vi "signal-NetVar-publisher.vi"() -> ()   [LabVIEW 2020]
uses:
  <vilib>/measure/NI_MABase.lvlib
panel:
  in  "Cluster":cluster{"Sampling Freq":dbl, "Samples":dbl}
  in  "Signal type":u16(ring) items=["Sine Wave", "Triangle Wave", "Square Wave", "Sawtooth Wave"]
  in  "Czestotliwosc":dbl(knob) scale=0.01..500.0
  in  "Amplituda":dbl(knob) scale=0.01..10.0
  in  "stop":bool
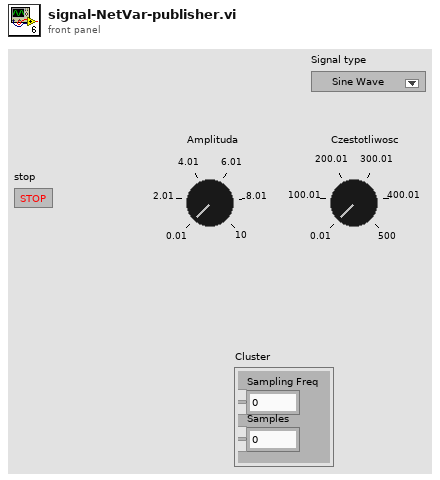
[diagram p1: front panel]
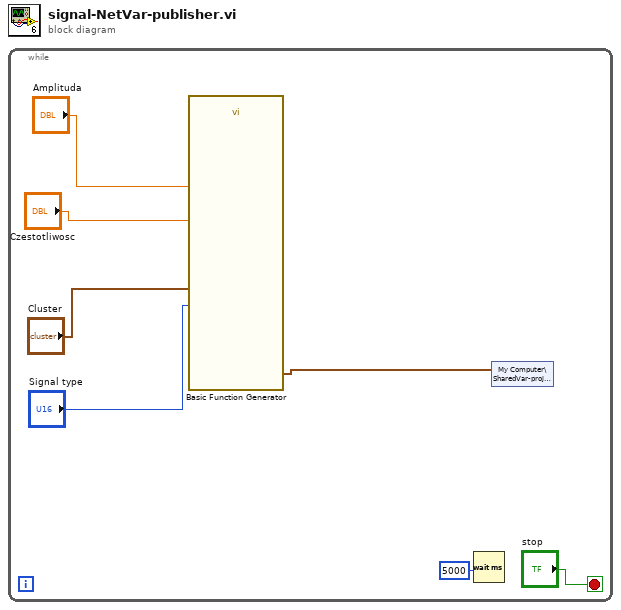
[diagram p0: block diagram]
diagram:
  n1 = while {
    stop <- "stop" stop-if-true
    n2 = call <vilib>:"Basic Function Generator.vi"("sampling info"="Cluster", "signal type"="Signal type", "amplitude"="Amplituda", "frequency"="Czestotliwosc") -> ("signal out"=w1:waveform(dbl))  [unwired: 5 in, 2 out]
    n3 = Wait (ms)(milliseconds to wait=5000) -> ()  [unwired: 1 out]
    n4 = shared-variable "My Computer\\SharedVar-project.lvlib\\Var"(w1) -> ()  [unwired: 1 in, 1 out]
  }
